vi "SQL READ DATA.vi"(8 "error out 2":errorcluster, 10 "Barcode":string="QWERTY", 11 "connection reference":T1) -> (0 "error out":errorcluster, 2 "Station1_Rst":string, 3 "connection reference out":T1)   [LabVIEW 2017]
uses:
  <vilib>/addons/database/Connection.llb/Conn ObjectReference.ctl
  <vilib>/addons/database/NI_Database_API.lvlib
panel:
  out "subarray":string[](array[string])
  out "no data":bool
  out "data 2":string[][](array[string])
  out "data":variant[][](array[variant])
  # "SEARCH FOR BARCODE DONE IN STATION1 AND RRSULT"
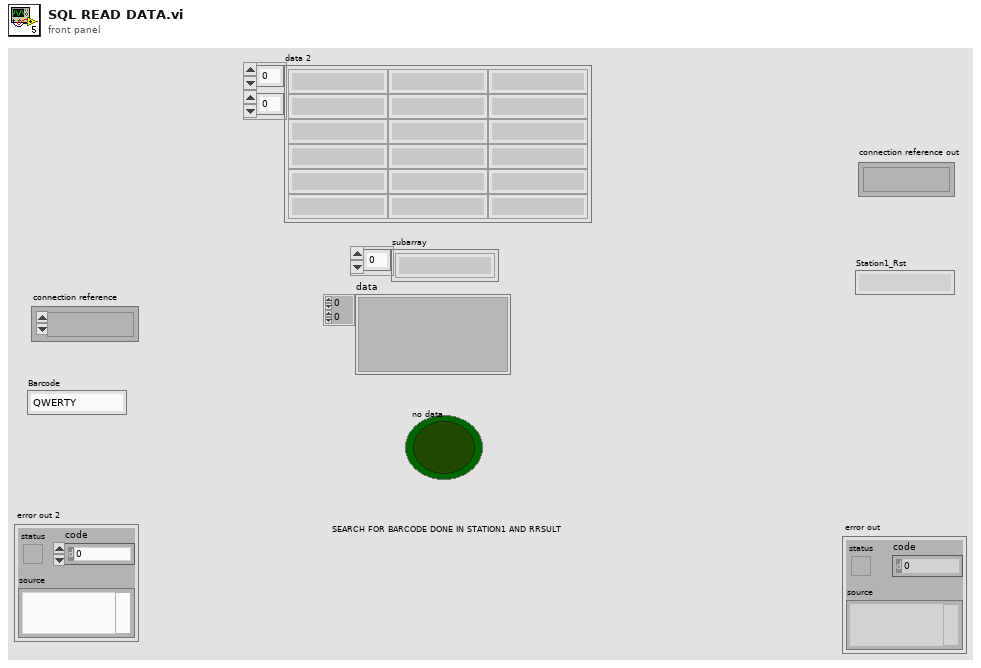
[diagram p1: front panel]
types:
  T1 = typedef "NI_Database_API.lvlib/Conn ObjectReference.ctl" = refnum<k1>
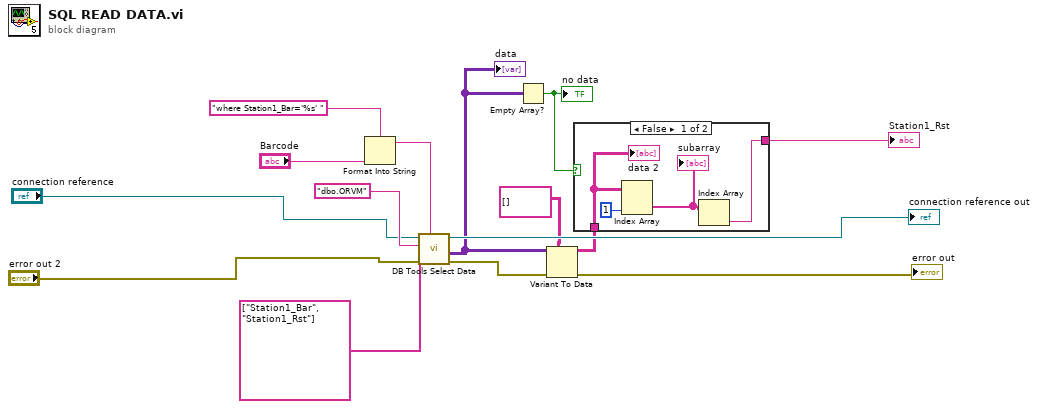
[diagram p0: block diagram]
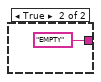
[diagram p2: hidden frame]
diagram:
  n1 = Format Into String(format string="where Station1_Bar='%s' ", "Barcode") -> (resulting string=w14:string)  [unwired: 2 in, 1 out]
  n2 = call <vilib>:"DB Tools Select Data.vi"("condition"=w14, "error in (no error)"="error out 2", "columns"=string[] ["Station1_Bar", "Station1_Rst"] ("columns 2"), "table"="dbo.ORVM", "connection reference"="connection reference") -> ("error out"=w8:errorcluster, "data"=w9:variant[][], "connection reference out"=→"connection reference out":T1)  [unwired: 1 in]
  "data" <- w9
  n3 = Empty Array?(array=w9) -> (empty?=w1:bool)
  "no data" <- w1
  n4 = Variant To Data(error in=w8, type=string[][] [], Variant=w9) -> (data=w6:string[][], error out=→"error out":errorcluster)
  n5 = case shown="False" w1 {
    tunnel: w6 -> [w19 _]
    tunnel: [w16 "EMPTY"] -> w5
    frame False {
      n6 = Index Array(array=w19, index (col)=1 ("disabled index (col)")) -> (element=w17:string[])  [unwired: 1 in]
      "subarray" <- w17
      n7 = Index Array(array=w17) -> (element=w16:string)  [unwired: 1 in]
      "data 2" <- w19
    }
    frame True {
    }
  }
  "Station1_Rst" <- w5
